vi "AddBus.vi"(9 "BusRef":refnum<vi>, 10 "BusNumberRef":refnum<vi>, 11 "BusArray":refnum<class "Bus.lvclass">[](array[class])) -> (3 "BusArray":refnum<class "Bus.lvclass">[](array[class]))   [LabVIEW 2017, in "Visualization.lvlib" / "VisualizeBase_class.lvclass"]
uses:
  VisializeBase_class/VisualizeBase_class.lvclass
  Framework/Bus_class/Bus.lvclass
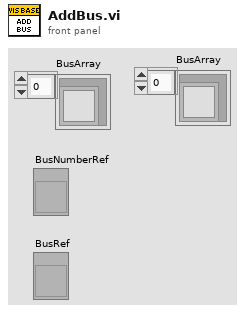
[diagram p1: front panel]
types:
  T1 = typedef "LVStringsAndValuesArrayTypeDef_U8.ctl" = cluster{"String":string, "Value":u8}[]
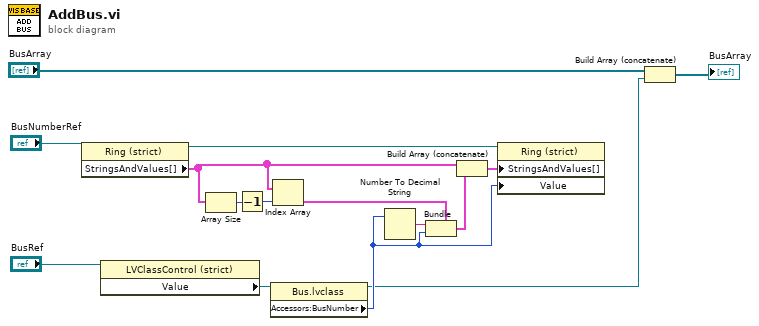
[diagram p0: block diagram]
diagram:
  n1 = property class="Ring (strict)"(reference="BusNumberRef") -> (reference out=w13:refnum<vi>, "StringsAndValues[]"=w14:T1)  [unwired: 1 in, 1 out]
  n2 = property class="LVClassControl (strict)"(reference="BusRef") -> ("Value"=w6:refnum<class "Bus.lvclass">)  [unwired: 1 in, 2 out]
  n3 = Array Size(array=w14) -> (size(s)=w9:i32)
  n4 = Decrement(x=w9) -> (x-1=w12:i32)
  n5 = property class="Bus.lvclass"(reference=w6) -> (reference out=w3:refnum<class "Bus.lvclass">, "Accessors:BusNumber"=w15:u8)  [unwired: 1 in, 1 out]
  n6 = Index Array(array=w14, index=w12) -> (element=w10:cluster{"String":string, "Value":u8})
  n7 = Number To Decimal String(number=w15) -> (decimal integer string=w7:string)  [unwired: 1 in]
  n8 = Bundle(cluster=w10, "String"=w7, "Value"=w15) -> (w11:cluster{"String":string, "Value":u8})
  n9 = Build Array (concatenate)(w14, w11) -> (w8:T1)
  n10 = property class="Ring (strict)"(reference=w13, "StringsAndValues[]"=w8, "Value"=w15) -> ()  [unwired: 1 in, 2 out]
  n11 = Build Array (concatenate)("BusArray", w3) -> (→"BusArray":refnum<class "Bus.lvclass">[])
